vi "DatabseTest.vi"() -> ()   [LabVIEW 2015]
uses:
  <vilib>/Utility/miscctls.llb/LVDateTimeRec.ctl
  DatabaseManager/DBManager.lvclass
panel:
  out "error out":errorcluster
  out "date time rec":T1
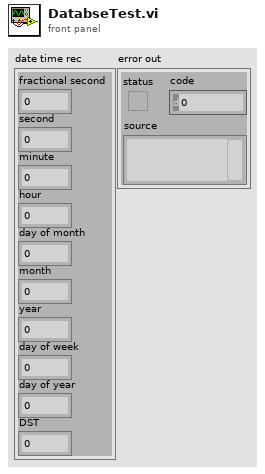
[diagram p1: front panel]
types:
  T1 = typedef "LVDateTimeRec.ctl" = cluster{"fractional second":dbl, "second":i32, "minute":i32, "hour":i32, "day of month":i32, "month":i32, "year":i32, "day of week":i32, "day of year":i32, "DST":i32}
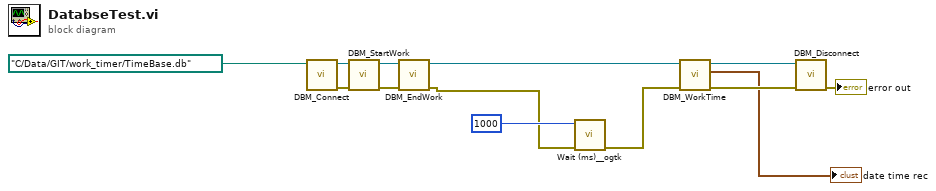
[diagram p0: block diagram]
diagram:
  n1 = call "DBM_Connect.vi"("Path"=path "C:/Data/GIT/work_timer/TimeBase.db") -> ("error out"=w12:errorcluster, "DBManager out"=w13:refnum<class "DBManager.lvclass">)  [unwired: 9 in]
  n2 = call "DBM_StartWork.vi"("error in (no error)"=w12, "DBManager in"=w13) -> ("error out"=w3:errorcluster, "DBManager out"=w4:refnum<class "DBManager.lvclass">)  [unwired: 8 in]
  n3 = call "DBM_EndWork.vi"("error in (no error)"=w3, "DBManager in"=w4) -> ("error out"=w1:errorcluster, "DBManager out"=w2:refnum<class "DBManager.lvclass">)  [unwired: 8 in]
  n4 = call <userlib>:"Wait (ms)__ogtk.vi"("error in (no error)"=w1, "milliseconds to wait"=u32 1000) -> ("error out"=w8:errorcluster)  [unwired: 8 in, 1 out]
  n5 = call "DBM_WorkTime.vi"("error in (no error)"=w8, "DBManager in"=w2) -> ("error out"=w10:errorcluster, "date time rec"=→"date time rec":T1, "DBManager out"=w11:refnum<class "DBManager.lvclass">)  [unwired: 7 in]
  n6 = call "DBM_Disconnect.vi"("error in (no error)"=w10, "DBManager in"=w11) -> ("error out"=→"error out":errorcluster)  [unwired: 9 in]
